vi "Progress_Increment.vi"(2 "error in (sync)":errorcluster, 3 "Dependency Source in":refnum<class "Dependency Source.lvclass">) -> (0 "Abort?":bool, 1 "Dependency Source out":refnum<class "Dependency Source.lvclass">)   [LabVIEW 2019, in "Project.Dependencies Finder.lvlib" / "Dependency Source.lvclass"]
uses:
  Dependency Source.lvclass
  Dependency Source.lvclass/Dependency Source.ctl
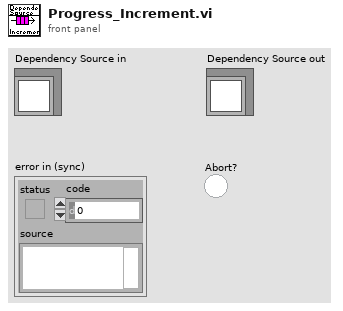
[diagram p1: front panel]
types:
  T1 = typedef "Project.Dependencies Finder.lvlib/Ctl_Progress Queue.ctl" = refnum<queue>
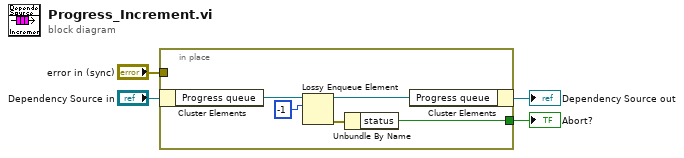
[diagram p0: block diagram]
diagram:
  n1 = in-place {
    in-place-border: [w5] -> w2
    in-place-border: "error in (sync)" -> [_]
    n2 = in-place-cluster #1("Dependency Source in") -> ("Progress queue"=w9:T1)
    n3 = Lossy Enqueue Element(queue=w9, element=-1) -> (queue out=w8:T1, error out=w6:errorcluster)  [unwired: 1 in, 2 out]
    n4 = Unbundle By Name(w6) -> ("status"=w5:bool)
    n5 = in-place-cluster #1("Progress queue"=w8) -> (→"Dependency Source out":refnum<class "Dependency Source.lvclass">)
  }
  "Abort?" <- w2
